vi "Launch OldLabActor.vi"() -> ()   [LabVIEW 2016]
uses:
  OldLabActor Class/OldLabActor.lvclass
  C:/github/LabActor/Controllers/Application Controller/Application Controller.lvclass
  Controllers/Application Controller/Load App.vi
  Controllers/Application Controller/Application Controller.lvclass
panel:
  out "Waiting Lights":T1
  out "Current action:":string
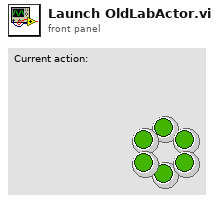
[diagram p1: front panel]
types:
  T1 = cluster{"DNL_wait 1":bool, "DNL_wait 1":bool, "DNL_wait 1":bool, "DNL_wait 1":bool, "DNL_wait 1":bool, "DNL_wait 1":bool}
  T2 = cluster{"[0]":bool, "[1]":bool, "[2]":bool, "[3]":bool, "[4]":bool, "[5]":bool}
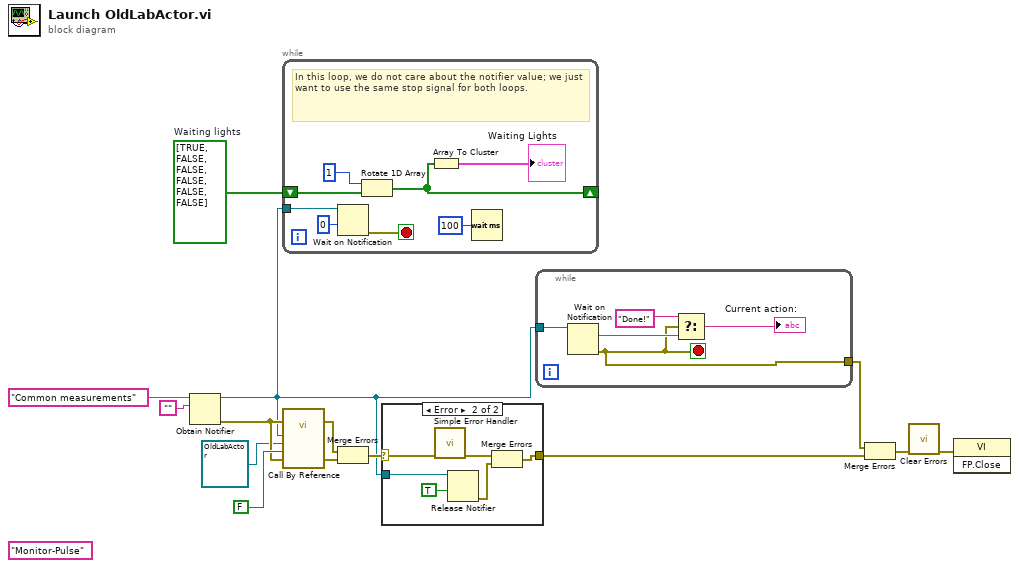
[diagram p0: block diagram]
diagram:
  (unwired) "Monitor-Pulse" ("Name")
  w3 = bool[] [TRUE, FALSE, FALSE, FALSE, FALSE, FALSE]  # Waiting lights
  n1 = Obtain Notifier(name (unnamed)="Common measurements", notification data type="") -> (notifier out=w1:refnum<notifier>, error out=w9:errorcluster)  [unwired: 2 in, 1 out]
  n2 = while {
    shift-right: [w16] -> _
    shift-left: w3 -> [w18]
    tunnel: w1 -> [w20]
    stop <- w22 stop-if-true
    # "In this loop, we do not care about the notifier value; we just want to use the same stop signal for both loops."
    n3 = Wait on Notification(notifier=w20, timeout in ms (-1)=0) -> (error out=w22:errorcluster)  [unwired: 2 in, 3 out]
    n4 = Rotate 1D Array(1:w18, 2:1 ("n")) -> (0:w16:bool[])
    n5 = Array To Cluster(array=w16) -> (cluster=→"Waiting Lights":T2)
    n6 = Wait (ms)(milliseconds to wait=u32 100) -> ()  [unwired: 1 out]
  }
  n7 = call-by-ref "?"(error in=w9, "Error In"=w9, "Open Actor Core front panel? (F)"=FALSE, "Application Controller.lvclass"=refnum<class "OldLabActor.lvclass"> refnum ("OldLabActor.lvclass"), "Status Notifier"=w1) -> (error out=w12:errorcluster, "Error Out"=w8:errorcluster)  [unwired: 8 in, 1 out]
  n8 = Merge Errors(w12, w8) -> (w13:errorcluster)
  n9 = case shown="Error" w13 {
    selector: w13 -> [w23 w29]
    tunnel: [w23 w25] -> w6
    tunnel: w1 -> [_ w26]
    frame No Error {
    }
    frame Error {
      n10 = call <vilib>:"Simple Error Handler.vi"("error in (no error)"=w29) -> ("error out"=w28:errorcluster)  [unwired: 4 in, 4 out]
      n11 = Release Notifier(notifier=w26, force destroy? (F)=TRUE ("Kill notifier")) -> (error out=w24:errorcluster)  [unwired: 1 in, 2 out]
      n12 = Merge Errors(w28, w24) -> (w25:errorcluster)
    }
  }
  n13 = while {
    tunnel: w1 -> [w34]
    tunnel: [w30] -> w4
    stop <- w30 stop-if-true
    n14 = Wait on Notification(notifier=w34) -> (notification=w32:string, error out=w30:errorcluster)  [unwired: 3 in, 2 out]
    n15 = Select(t="Done!" ("notification"), s=w30, f=w32) -> (s? t:f=→"Current action:":string)
  }
  n16 = Merge Errors(w4, w6) -> (w5:errorcluster)
  n17 = call <vilib>:"Clear Errors.vi"("error in (no error)"=w5) -> ("error out"=w14:errorcluster)  [unwired: 5 in, 1 out]
  n18 = invoke class="VI" method="FP.Close"(error in=w14) -> ()  [unwired: 2 in, 3 out]
